vi "Build Parameters.vi"(10 "Scenarios In":cluster{"Scenario":string, "Parameters":T2}[](array[cluster])) -> (2 "Scenarios out":T1(array[cluster]))   [LabVIEW 2020, in "test.lvlib" / "02_FeatureDetectionAprilTag.lvclass"]
doc: "This helper function simplifies the syntax of creating parameters."
uses:
  02_FeatureDetectionAprilTag.lvclass
  Parameters.ctl
  common/Image Point (Float).ctl
  common/Square Corners.ctl
  02_FeatureDetectionAprilTag.lvclass/02_FeatureDetectionAprilTag.ctl
  common/common.lvlib
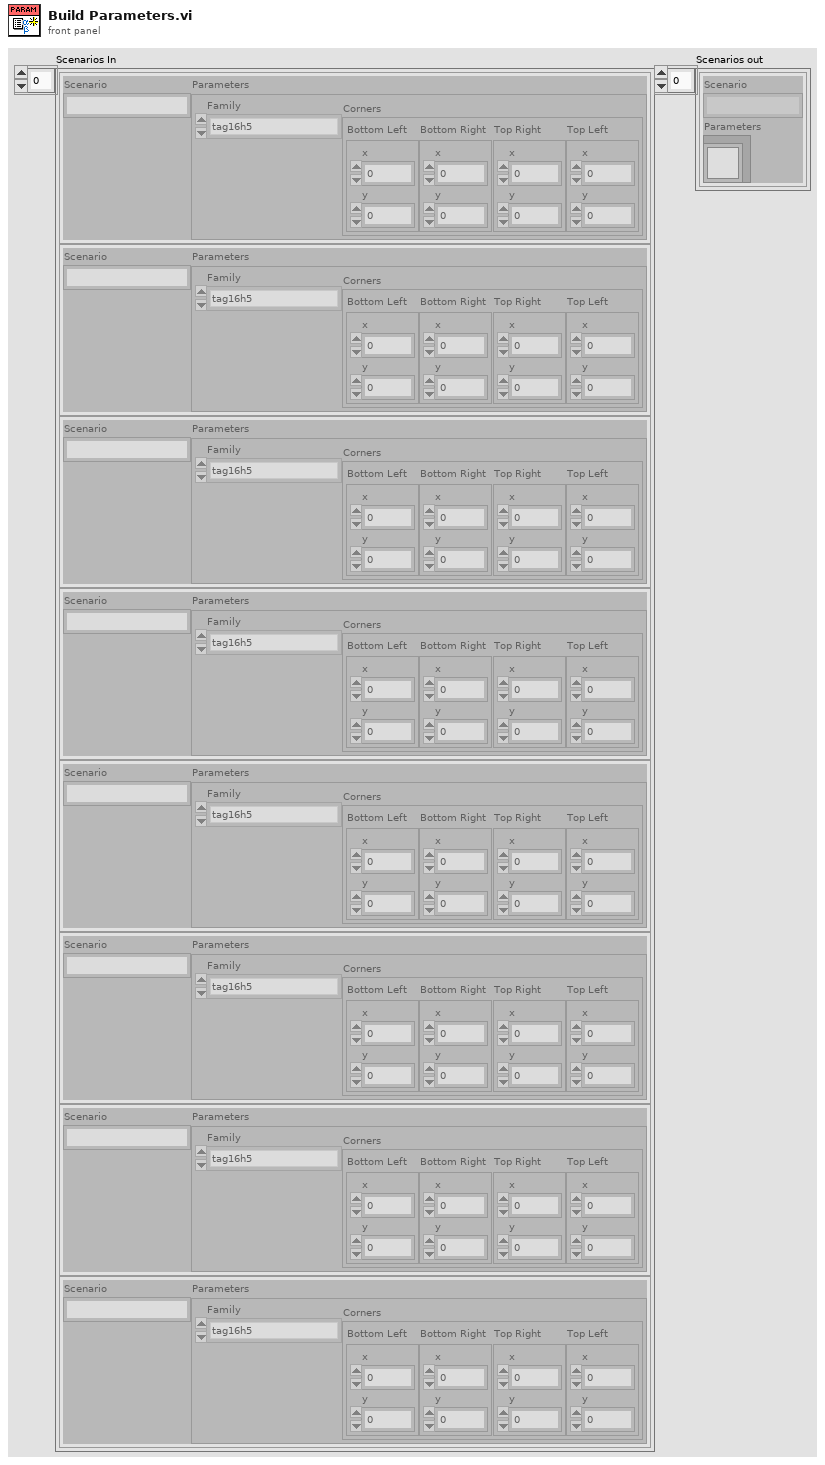
[diagram p1: front panel]
types:
  T1 = cluster{"Scenario":string, "Parameters":refnum<class "02_FeatureDetectionAprilTag.lvclass">}[]
  T2 = typedef "test.lvlib/02_FeatureDetectionAprilTag.lvclass/Parameters.ctl" = cluster{"Family":enum8{"tag16h5", "tag25h9", "tag36h11", "tagCircle21h7", "tagCircle49h12", "tagCustom48h12", "tagStandard41h12", "tagStandard52h13"}, "Corners":T3}
  T3 = typedef "common.lvlib/Square Corners.ctl" = cluster{"Bottom Left":T4, "Bottom Right":T4, "Top Right":T4, "Top Left":T4}
  T4 = typedef "common.lvlib/Image Point (Float).ctl" = cluster{"x":dbl, "y":dbl}
  T5 = cluster{"Scenario":string, "Parameters":refnum<class "02_FeatureDetectionAprilTag.lvclass">}
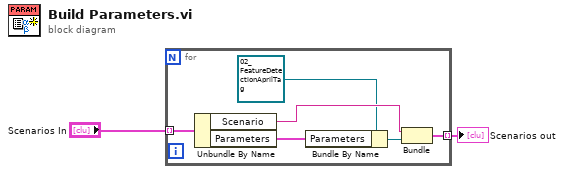
[diagram p0: block diagram]
diagram:
  n1 = for {
    tunnel: [w4] -> w1 mode=indexing
    tunnel: "Scenarios In" -> [w8] mode=indexing
    n2 = Unbundle By Name(w8) -> ("Scenario"=w7:string, "Parameters"=w3:T2)
    n3 = Bundle By Name(cluster=refnum<class "02_FeatureDetectionAprilTag.lvclass"> refnum ("Parameters"), "Parameters"=w3) -> (w5:refnum<class "02_FeatureDetectionAprilTag.lvclass">)
    n4 = Bundle("Scenario"=w7, "Parameters"=w5) -> (w4:T5)  [unwired: 1 in]
  }
  "Scenarios out" <- w1
